vi "VorC.vi"(8 "Buf":sgl[][](array[numeric]), 11 "电压电流选择":enum32{"单选选项1", "单选选项2"}(radio)) -> (2 "Buf 2":sgl[][](array[numeric]))   [LabVIEW 2016]
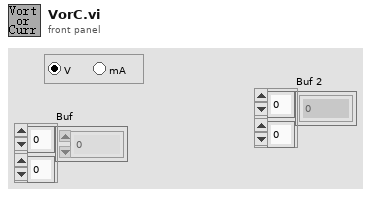
[diagram p1: front panel]
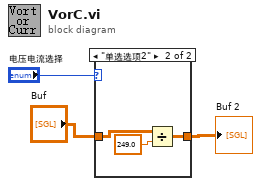
[diagram p0: block diagram]
diagram:
  n1 = case shown="\"单选选项2\"" "电压电流选择" {
    tunnel: "Buf" -> [w4 w6]
    tunnel: [w4 w5] -> w1
    frame "单选选项1", Default {
    }
    frame "单选选项2" {
      n2 = Divide(x=w6, y=249.0) -> (x/y=w5:dbl[][])
    }
  }
  "Buf 2" <- w1
